vi "Get Name.vi"(8 "error in (no error)":errorcluster, 11 "PropertyObject in":refnum<class "PropertyObject.lvclass">) -> (0 "error out":errorcluster, 2 "Name":string, 3 "PropertyObject out":refnum<class "PropertyObject.lvclass">)   [LabVIEW 2020, in "TSnax.lvlib" / "PropertyObject.lvclass"]
uses:
  PropertyObject.lvclass
  PropertyObject.lvclass/PropertyObject.ctl
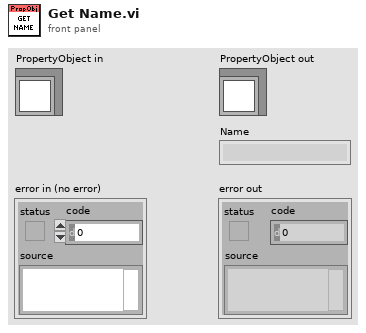
[diagram p1: front panel]
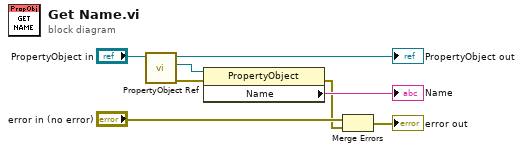
[diagram p0: block diagram]
diagram:
  n1 = call "PropertyObject Ref.vi"("PropertyObject in"="PropertyObject in") -> ("error out"=w4:errorcluster, "PropertyObject"=w7:refnum<k7>, "PropertyObject out"=→"PropertyObject out":refnum<class "PropertyObject.lvclass">)  [unwired: 8 in]
  n2 = property class="PropertyObject"(reference=w7, error in=w4) -> (error out=w1:errorcluster, "Name"=→"Name":string)  [unwired: 1 out]
  n3 = Merge Errors("error in (no error)", w1) -> (→"error out":errorcluster)
